vi "GetFirstNotFullLibrary.vi"(8 "error in (no error)":errorcluster, 10 "LibraryName":string, 11 "Connection in":refnum<class "Connection.lvclass">) -> (0 "error out":errorcluster, 1 "Result":T1, 2 "Valid":bool, 3 "Connection out":refnum<class "Connection.lvclass">)   [LabVIEW 2018, in "ErrorDefinitionSQLite.lvclass"]
uses:
  ErrorDefinitionSQLite.lvclass
  <vilib>/drjdpowell/SQLite Library/SQL Connection/Connection.lvclass
  <vilib>/drjdpowell/SQLite Library/SQL Connection/Execute SQL.vi
  <vilib>/drjdpowell/SQLite Library/SQLite.lvlib
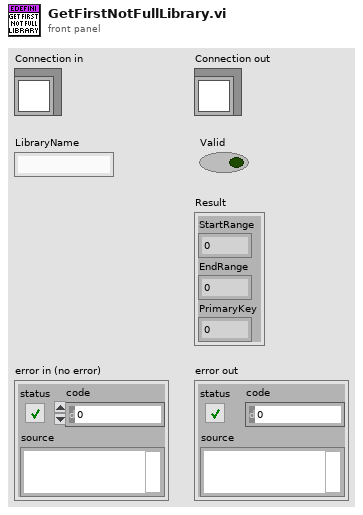
[diagram p1: front panel]
types:
  T1 = cluster{"StartRange":i32, "EndRange":i32, "PrimaryKey":i32}
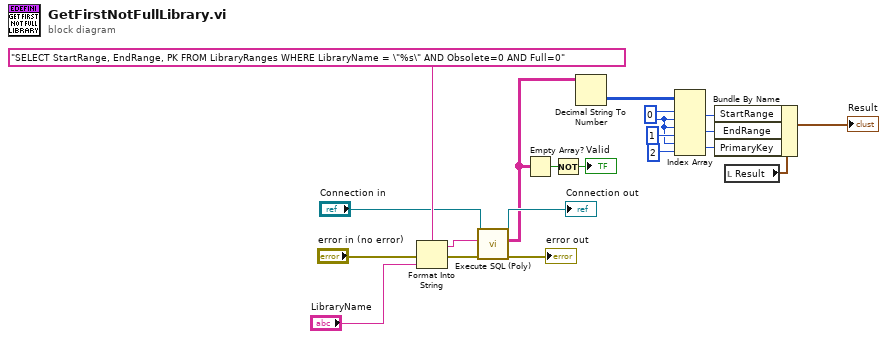
[diagram p0: block diagram]
diagram:
  w9 = 0 ("disabled index (col)")
  n1 = Format Into String(format string="SELECT StartRange, EndRange, PK FROM LibraryRanges WHERE LibraryName = \"%s\" AND Obsolete=0 AND Full=0" ("SQL"), error in="error in (no error)", "LibraryName") -> (resulting string=w17:string, error out=w14:errorcluster)  [unwired: 1 in]
  n2 = call-poly <vilib>:"Execute SQL (Poly).vi"("error in (no error)"=w14, "SQL"=w17, "SQLite Connection in"="Connection in") -> ("error out"=→"error out":errorcluster, "Result Set"=w7:string[][], "SQLite Connection"=→"Connection out":refnum<class "Connection.lvclass">)  [unwired: 5 in, 1 out]
  n3 = Empty Array?(array=w7) -> (empty?=w20:bool)
  n4 = Not(x=w20) -> (.not. x?=→"Valid":bool)
  n5 = Decimal String To Number(string=w7) -> (number=w6:i32[][])  [unwired: 2 in, 1 out]
  n6 = Index Array(array=w6, index (row) #1=w9, index (col) #1=w9, index (row) #2=w9, index (col) #2=1 ("disabled index (row)"), index (row) #3=w9, index (col) #3=2 ("disabled index (row)")) -> (element #1=w5:i32, element #2=w4:i32, element #3=w3:i32)
  n7 = local read "Result"() -> (w1:T1)
  n8 = Bundle By Name(cluster=w1, "StartRange"=w5, "EndRange"=w4, "PrimaryKey"=w3) -> (→"Result":T1)
